vi "OA Get Number Of Acq Params.vi"(8 "error in (no error)":errorcluster, 10 "puiNumberOfParams":u32, 11 "pcModeName":string) -> (0 "error out":errorcluster, 2 "puiNumberOfParams out":u32, 3 "function return":u32)   [LabVIEW 2014, in "atmcd32d.lvlib"]
doc: "unsigned int WINAPI OA_GetNumberOfAcqParams(const char * const pcModeName, unsigned int * const puiNumberOfParams);"
uses:
  atmcd32d.lvlib
  atmcd32d.dll
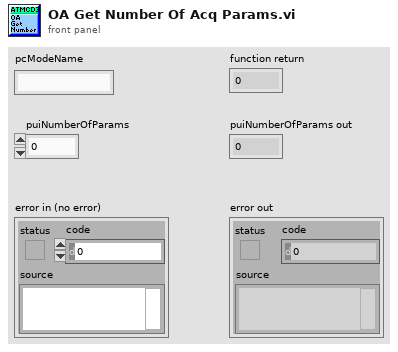
[diagram p1: front panel]
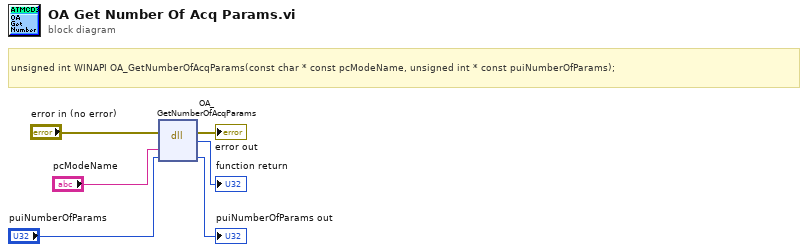
[diagram p0: block diagram]
diagram:
  # "unsigned int WINAPI OA_GetNumberOfAcqParams(const char * const pcModeName, unsigned int * const puiNumberOfParams);"
  n1 = dll-call lib="C:/Users/Bakir/Documents/Lambda2-Testing/lib/Andorlib/atmcd32d.*" fn="OA_GetNumberOfAcqParams"(error in="error in (no error)", "pcModeName"="pcModeName", "puiNumberOfParams"="puiNumberOfParams") -> (error out=→"error out":errorcluster, →"function return":u32, "puiNumberOfParams"=→"puiNumberOfParams out":u32)  [unwired: 3 in, 1 out]
